vi "Flush LogMeasData Q.vi"(8 "error in (no error)":errorcluster) -> (0 "error out":errorcluster, 1 "Remaining MeasData[] out":T1[](array[typedef]), 3 "orData out":T4)   [LabVIEW 2019]
doc: "Developed by Kevin Thompson\nThompson Engineering, LLC\nkevin@thompsonengineering.net"
uses:
  TD MeasData--cluster.ctl
  TD MeasData QRef.ctl
  GBL DataQ Ref.vi
  DataTypes/InverterData--cluster.ctl
  DataTypes/InverterPhaseData--cluster.ctl
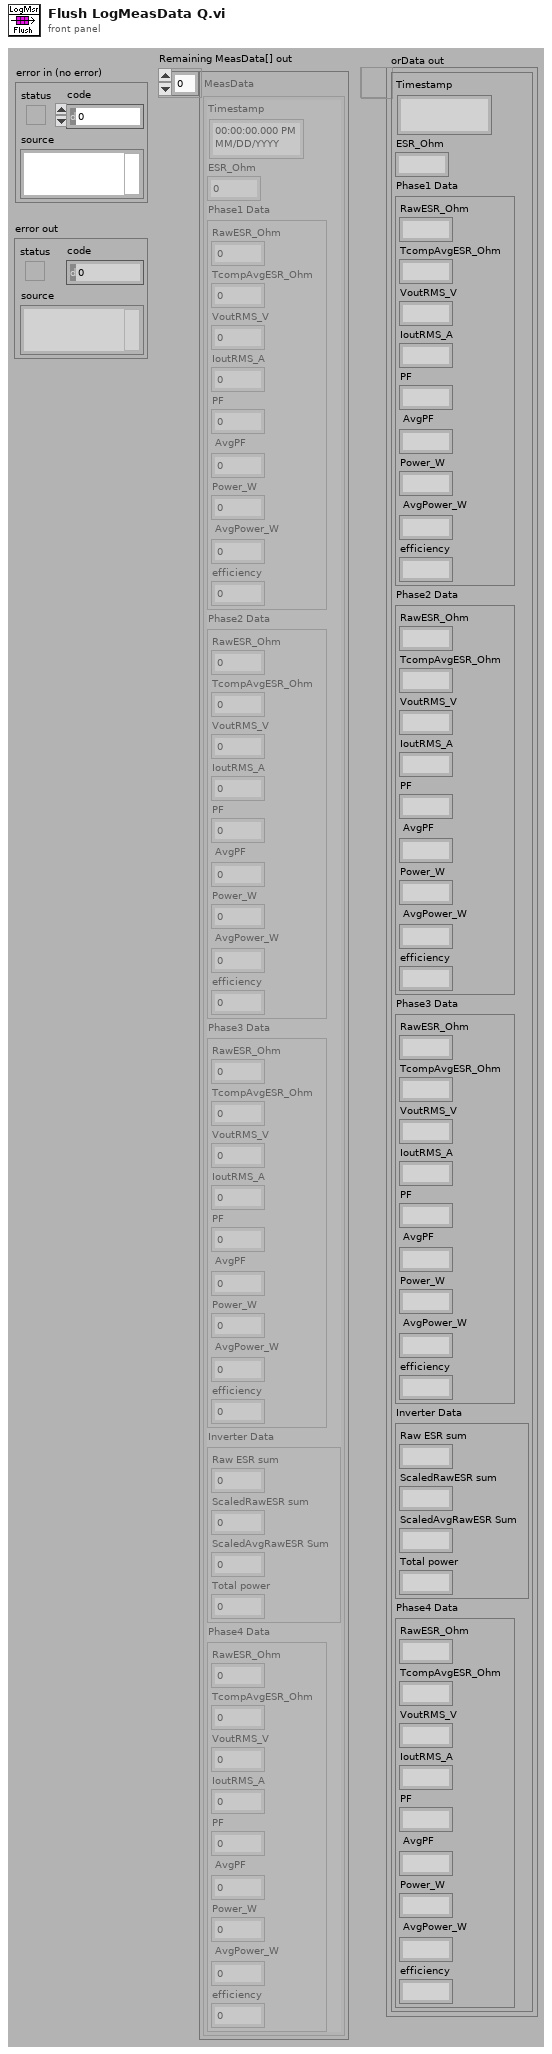
[diagram p1: front panel]
types:
  T1 = typedef "TD MeasData--cluster.ctl" = cluster{"Timestamp":timestamp, "ESR_Ohm":dbl, "Phase1 Data":T2, "Phase2 Data":T2, "Phase3 Data":T2, "Inverter Data":T3, "Phase4 Data":T2}
  T2 = typedef "InverterPhaseData--cluster.ctl" = cluster{"RawESR_Ohm":dbl, "TcompAvgESR_Ohm":dbl, "VoutRMS_V":dbl, "IoutRMS_A":dbl, "PF":dbl, "AvgPF":dbl, "Power_W":dbl, "AvgPower_W":dbl, "efficiency":dbl}
  T3 = typedef "InverterData--cluster.ctl" = cluster{"Raw ESR sum":dbl, "ScaledRawESR sum":dbl, "ScaledAvgRawESR Sum":dbl, "Total power":dbl}
  T4 = typedef "TD MeasData QRef.ctl" = refnum<queue>
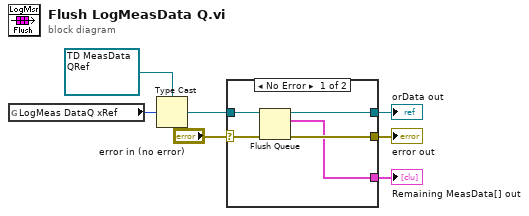
[diagram p0: block diagram]
diagram:
  n1 = global read "GBL DataQ Ref.vi" "LogMeas DataQ xRef"() -> (w1:u32)
  n2 = Type Cast(type=T4 refnum ("MeasDataQRef"), x=w1) -> (*(type *) &x=w4:T4)
  n3 = case shown="No Error" "error in (no error)" {
    selector: "error in (no error)" -> [w9 w13]
    tunnel: w4 -> [w10 w14]
    tunnel: [w12 w13] -> w7
    tunnel: [w11 w14] -> w6
    tunnel: [w8 _] -> w3
    frame No Error {
      n4 = Flush Queue(queue=w10, error in (no error)=w9) -> (queue out=w11:T4, remaining elements=w8:T1[], error out=w12:errorcluster)
    }
    frame Error {
    }
  }
  "orData out" <- w6
  "error out" <- w7
  "Remaining MeasData[] out" <- w3
